vi "Get Device Properties.vi"(8 "error in (no error)":errorcluster, 11 "Custom Device":refnum<k24>) -> (0 "error out":errorcluster, 1 "Decimation":i32=1, 2 "VISA Name":string, 3 "Custom Device Duplicate":refnum<k24>, 5 "CPU Assignment":i32=-2)   [LabVIEW 2010, in "RefMem PtByPt System Definition API.lvlib"]
doc: "Set the VISA name and Decimation of the custom device."
uses:
  RefMem PtByPt System Definition API.lvlib
  NationalInstruments.VeriStand.SystemDefinitionAPI
  Custom Device/Controls/Global.vi
  Custom Device/RefMem PtByPt Custom Device.lvlib
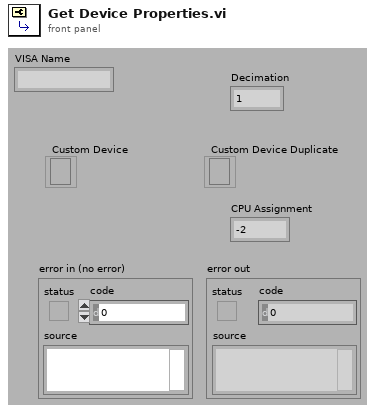
[diagram p1: front panel]
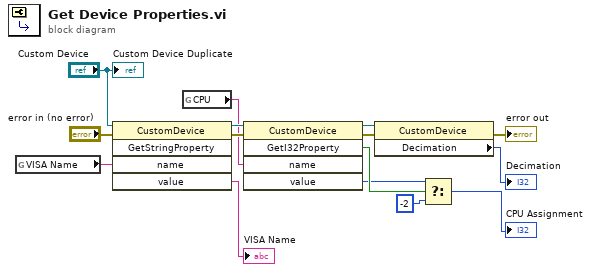
[diagram p0: block diagram]
diagram:
  n1 = global read "Global.vi" "VISA Name"() -> (w13:string)
  n2 = invoke class="CustomDevice" method="GetStringProperty"(reference="Custom Device", error in="error in (no error)", "name"=w13) -> (reference out=w10:refnum<k24>, error out=w9:errorcluster, "value"=→"VISA Name":string)  [unwired: 2 in, 2 out]
  n3 = global read "Global.vi" "CPU"() -> (w8:string)
  n4 = invoke class="CustomDevice" method="GetI32Property"(reference=w10, error in=w9, "name"=w8) -> (reference out=w12:refnum<k24>, error out=w11:errorcluster, "GetI32Property"=w4:bool, "value"=w2:i32)  [unwired: 2 in, 1 out]
  n5 = property class="CustomDevice"(reference=w12, error in=w11) -> (error out=→"error out":errorcluster, "Decimation"=→"Decimation":i32)  [unwired: 1 out]
  n6 = Select(t=w2, s=w4, f=-2) -> (s? t:f=→"CPU Assignment":i32)
  "Custom Device Duplicate" <- "Custom Device"
